vi "FGV_SimpleNumeric.vi"(10 "Numeric":i32, 11 "Mode":enum16{"SET", "GET"}(ring)) -> (2 "Numeric Out":i32)   [LabVIEW 2020]
doc: "Example of GET/SET Functional Global Variabl with numeric data. Comments in Polish."
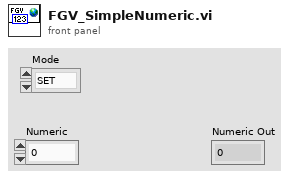
[diagram p1: front panel]
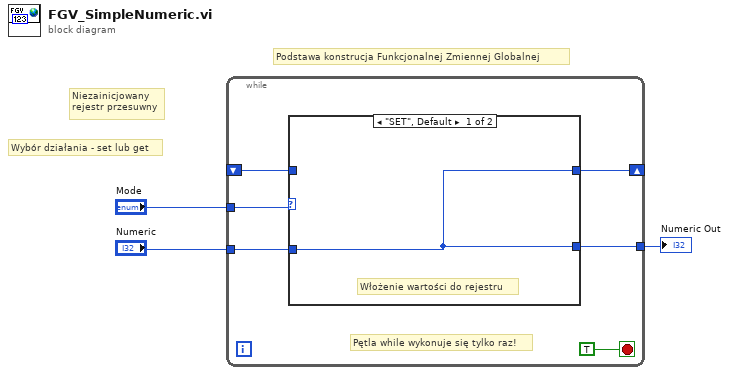
[diagram p0: block diagram]
diagram:
  # "Wybór działania - set lub get"
  # "Niezainicjowany\nrejestr przesuwny"
  # "Podstawa konstrucja Funkcjonalnej Zmiennej Globalnej"
  n1 = while {
    tunnel: "Mode" -> [w8]
    shift-right: [w6] -> _
    shift-left: _ -> [w4]
    tunnel: "Numeric" -> [w7]
    tunnel: [w5] -> w2
    stop <- TRUE stop-if-true
    # "Pętla while wykonuje się tylko raz!"
    n2 = case shown="\"SET\", Default" w8 {
      tunnel: w7 -> [w10 _]
      tunnel: [w10 w11] -> w6
      tunnel: [w10 w11] -> w5
      tunnel: w4 -> [_ w11]
      frame "SET", Default {
        # "Włożenie wartości do rejestru"
      }
      frame "GET" {
        # "Wyjęcie wartości do rejestru"
      }
    }
  }
  "Numeric Out" <- w2
